vi "NMEA to Degrees.vi"(11 "NMEA Input":dbl[](array[numeric]) format="%#_8g") -> (3 "Degrees Output":dbl[](array[numeric]) format="%#_9g")   [LabVIEW 2014]
panel:
  out "Numeric":dbl
  # "NMEA to Degrees Conversion"
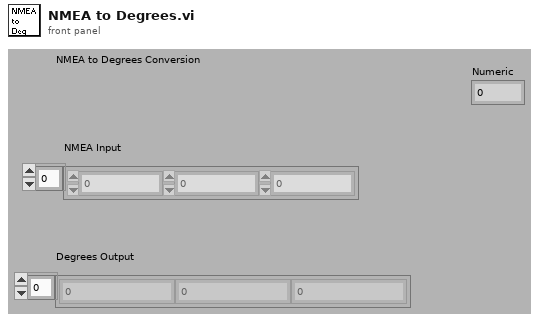
[diagram p1: front panel]
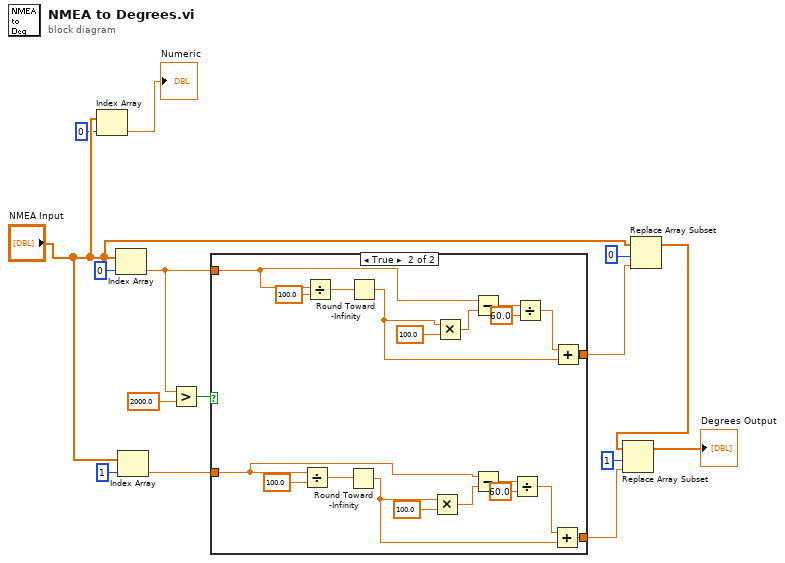
[diagram p0: block diagram]
diagram:
  n1 = Index Array(array="NMEA Input", index=0) -> (element=→"Numeric":dbl)
  n2 = Index Array(array="NMEA Input", index=0) -> (element=w5:dbl)
  n3 = Index Array(array="NMEA Input", index=1) -> (element=w8:dbl)
  n4 = Greater?(x=w5, y=2000.0) -> (0:w6:bool)
  n5 = case shown="True" w6 {
    tunnel: w5 -> [w16 w35]
    tunnel: [w16 w28] -> w11
    tunnel: w8 -> [w17 w23]
    tunnel: [w17 w18] -> w7
    frame False {
    }
    frame True {
      n6 = Divide(x=w23, y=100.0) -> (x/y=w26:dbl)
      n7 = Divide(x=w35, y=100.0) -> (x/y=w36:dbl)
      n8 = Round Toward -Infinity(1:w26) -> (0:w19:dbl)
      n9 = Round Toward -Infinity(1:w36) -> (0:w29:dbl)
      n10 = Multiply(x=w19, y=100.0) -> (x*y=w24:dbl)
      n11 = Multiply(x=w29, y=100.0) -> (x*y=w34:dbl)
      n12 = Subtract(x=w35, y=w34) -> (x-y=w32:dbl)
      n13 = Subtract(x=w23, y=w24) -> (x-y=w22:dbl)
      n14 = Divide(x=w22, y=60.0) -> (x/y=w20:dbl)
      n15 = Divide(x=w32, y=60.0) -> (x/y=w30:dbl)
      n16 = Add(x=w20, y=w19) -> (x+y=w18:dbl)
      n17 = Add(x=w30, y=w29) -> (x+y=w28:dbl)
    }
  }
  n18 = Replace Array Subset(array="NMEA Input", new element=w11, index=0) -> (w10:dbl[])
  n19 = Replace Array Subset(array=w10, new element=w7, index=1) -> (→"Degrees Output":dbl[])
